vi "INI File Read Error.vi"(8 "error in (no error)":errorcluster, 11 "INI Key Not Found?":bool) -> (0 "error out":errorcluster)   [LabVIEW 2016, in "CD Parameter Manager API.lvlib" / "Parameter INI File.lvclass"]
uses:
  Parameter INI File.lvclass
  <vilib>/ErrorRing/Error Ring.xnode
  <vilib>/Utility/error.llb/Error Cluster From Error Code.vi
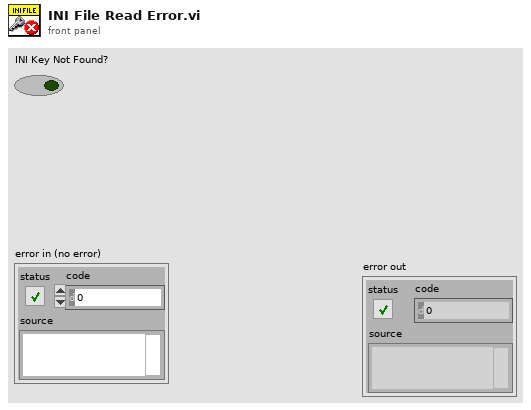
[diagram p1: front panel]
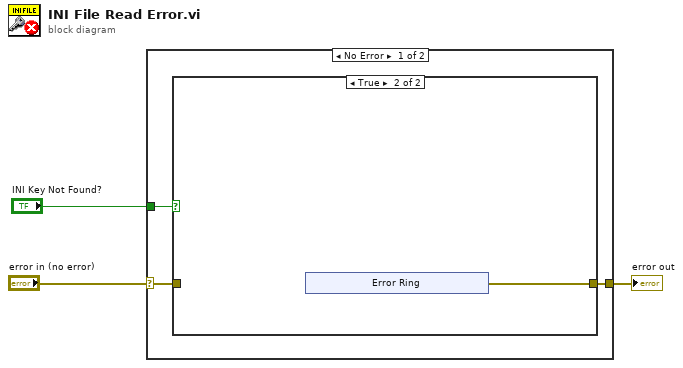
[diagram p0: block diagram]
diagram:
  n1 = case shown="No Error" "error in (no error)" {
    selector: "error in (no error)" -> [w6 w14]
    tunnel: [w5 w14] -> w2
    tunnel: "INI Key Not Found?" -> [w4 _]
    frame No Error {
      n2 = case shown="True" w4 {
        tunnel: [w7 w8] -> w5
        tunnel: w6 -> [w7 _]
        frame False {
        }
        frame True {
          n3 = xnode "Error Ring"() -> ("error out"=w8:errorcluster)
        }
      }
    }
    frame Error {
    }
  }
  "error out" <- w2
